vi "Set DDS Sweep Time.vi"(8 "error in (no error)":errorcluster, 10 "time_ns":u64, 11 "channel_index":u8) -> (0 "error out":errorcluster)   [LabVIEW 2021, in "vmmso.lvlib"]
doc: "DLL_API void WINAPI SetDDSSweepTime(unsigned char channel_index, unsigned long long int time_ns);"
uses:
  vmmso.lvlib
  vmmso.dll
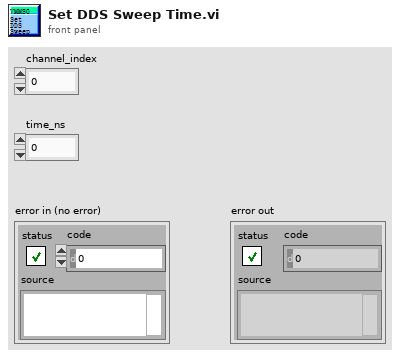
[diagram p1: front panel]
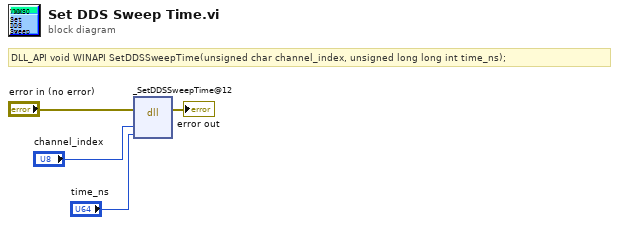
[diagram p0: block diagram]
diagram:
  # "DLL_API void WINAPI SetDDSSweepTime(unsigned char channel_index, unsigned long long int time_ns);"
  n1 = dll-call lib="O:/MSO/library/demo-Labview/vmmso/vmmso.*" fn="_SetDDSSweepTime@12"(error in="error in (no error)", "channel_index"="channel_index", "time_ns"="time_ns") -> (error out=→"error out":errorcluster)  [unwired: 5 in, 1 out]
